vi "test_libssh2_channel_forward_accept.vi"() -> ()   [LabVIEW 2013, in "libssh2_integration_tests.lvlib"]
uses:
  libssh2_integration_tests.lvlib
  <vilib>/addons/_JKI Toolkits/Caraya/classes/Test/Test.lvclass
  support/support.lvlib
  libssh2/libssh2.lvlib
  <vilib>/addons/_JKI Toolkits/Caraya/classes/Assert/Assert.lvclass
panel:
  out "error out":errorcluster
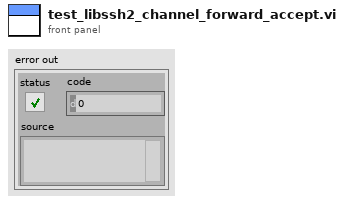
[diagram p1: front panel]
types:
  T1 = typedef "libssh2.lvlib/Session Refnum.ctl" = refnum<k1>
  T2 = typedef "libssh2.lvlib/Listener Refnum.ctl" = refnum<k1>
  T3 = typedef "libssh2.lvlib/Channel Refnum.ctl" = refnum<k1>
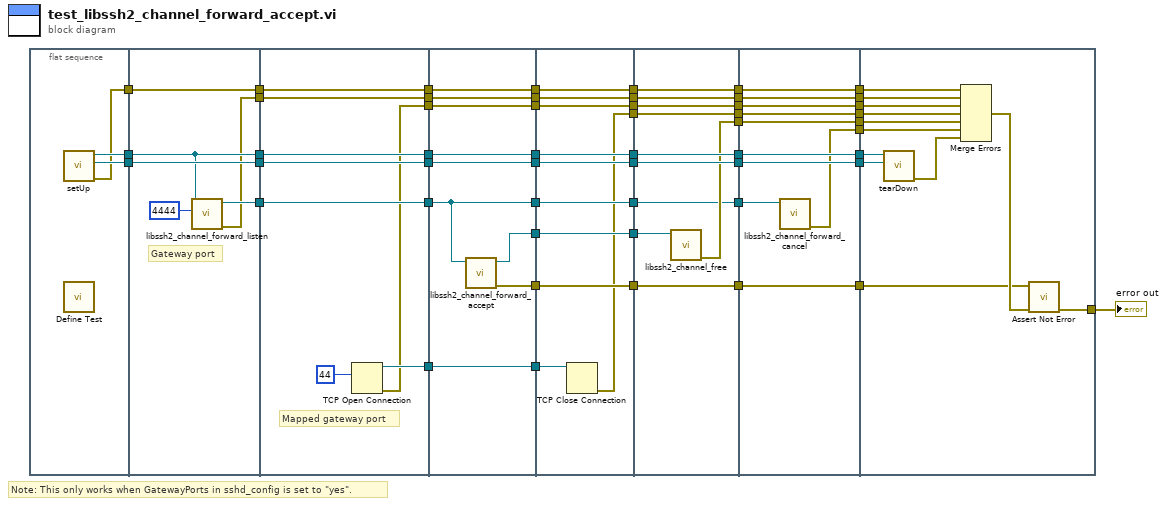
[diagram p0: block diagram]
diagram:
  # "Note: This only works when GatewayPorts in sshd_config is set to \"yes\"."
  n1 = flat-sequence {
    tunnel: [w55] -> w52
    tunnel: [w54] -> w51
    tunnel: [w53] -> w50
    tunnel: w52 -> [w59]
    tunnel: w51 -> [w61]
    tunnel: [w59] -> w33
    tunnel: [w61] -> w31
    tunnel: w50 -> [w60]
    tunnel: [w60] -> w29
    tunnel: [w57] -> w27
    tunnel: [w58] -> w25
    tunnel: w33 -> [w65]
    tunnel: [w65] -> w32
    tunnel: w31 -> [w69]
    tunnel: [w69] -> w30
    tunnel: w29 -> [w68]
    tunnel: [w68] -> w28
    tunnel: w27 -> [w67]
    tunnel: [w67] -> w26
    tunnel: w25 -> [w66]
    tunnel: [w66] -> w24
    tunnel: [w63] -> w23
    tunnel: [w62] -> w22
    tunnel: w32 -> [w78]
    tunnel: [w78] -> w43
    tunnel: w30 -> [w77]
    tunnel: [w77] -> w42
    tunnel: w28 -> [w76]
    tunnel: [w76] -> w41
    tunnel: w26 -> [w75]
    tunnel: [w75] -> w40
    tunnel: w24 -> [w74]
    tunnel: [w74] -> w39
    tunnel: [w73] -> w38
    tunnel: [w71] -> w37
    tunnel: [w72] -> w35
    tunnel: w23 -> [w71]
    tunnel: w22 -> [w70]
    tunnel: [w70] -> w21
    tunnel: w43 -> [w88]
    tunnel: w42 -> [w87]
    tunnel: [w88] -> w49
    tunnel: [w87] -> w48
    tunnel: [w84] -> w47
    tunnel: w41 -> [w86]
    tunnel: [w86] -> w46
    tunnel: w40 -> [w85]
    tunnel: [w85] -> w45
    tunnel: w39 -> [w81]
    tunnel: w38 -> [w84]
    tunnel: w37 -> [w82]
    tunnel: [w83] -> w36
    tunnel: w35 -> [w83]
    tunnel: [w81] -> w34
    tunnel: w21 -> [w80]
    tunnel: [w80] -> w20
    tunnel: [w79] -> w19
    tunnel: w49 -> [w98]
    tunnel: w48 -> [w97]
    tunnel: w47 -> [w96]
    tunnel: [w98] -> w18
    tunnel: [w97] -> w16
    tunnel: [w95] -> w14
    tunnel: w46 -> [w94]
    tunnel: [w94] -> w12
    tunnel: w45 -> [w93]
    tunnel: [w93] -> w10
    tunnel: [w92] -> w8
    tunnel: w36 -> [w92]
    tunnel: [w91] -> w6
    tunnel: w34 -> [w91]
    tunnel: w20 -> [w90]
    tunnel: [w90] -> w5
    tunnel: w19 -> [w89]
    tunnel: [w89] -> w3
    tunnel: w18 -> [w108]
    tunnel: [w108] -> w17
    tunnel: w16 -> [w107]
    tunnel: [w107] -> w15
    tunnel: w14 -> [w106]
    tunnel: [w106] -> w13
    tunnel: w12 -> [w105]
    tunnel: [w105] -> w11
    tunnel: w10 -> [w104]
    tunnel: [w104] -> w9
    tunnel: w8 -> [w103]
    tunnel: [w103] -> w7
    tunnel: w6 -> [w100]
    tunnel: w5 -> [w102]
    tunnel: [w102] -> w4
    tunnel: w3 -> [w101]
    tunnel: [w101] -> w2
    tunnel: [w99] -> w1
    tunnel: w17 -> [w120]
    tunnel: w15 -> [w119]
    tunnel: [w118] -> w44
    tunnel: w13 -> [w116]
    tunnel: w11 -> [w115]
    tunnel: w9 -> [w113]
    tunnel: w7 -> [w112]
    tunnel: w4 -> [w111]
    tunnel: w2 -> [w110]
    tunnel: w1 -> [w109]
    frame #0 {
      n2 = call "setUp.vi"() -> ("error out"=w53:errorcluster, "connection ID"=w54:refnum<k5>, "session"=w55:T1)  [unwired: 9 in]
      n3 = call <vilib>:"Define Test.vi"() -> ()  [unwired: 10 in, 2 out]
    }
    frame #1 {
      # "Gateway port"
      n4 = call "libssh2_channel_forward_listen.vi"("port in"=4444, "session"=w59) -> ("error out"=w57:errorcluster, "listener"=w58:T2)  [unwired: 7 in, 1 out]
    }
    frame #2 {
      # "Mapped gateway port"
      n5 = TCP Open Connection(remote port or service name=u16 44) -> (connection ID=w63:refnum<k5>, error out=w62:errorcluster)  [unwired: 4 in]
    }
    frame #3 {
      n6 = call "libssh2_channel_forward_accept.vi"("listener"=w74) -> ("error out"=w72:errorcluster, "channel"=w73:T3)  [unwired: 9 in]
    }
    frame #4 {
      n7 = TCP Close Connection(connection ID=w82) -> (error out=w79:errorcluster)  [unwired: 2 in, 1 out]
    }
    frame #5 {
      n8 = call "libssh2_channel_free.vi"("channel"=w96) -> ("error out"=w95:errorcluster)  [unwired: 10 in]
    }
    frame #6 {
      n9 = call "libssh2_channel_forward_cancel.vi"("listener"=w100) -> ("error out"=w99:errorcluster)  [unwired: 10 in]
    }
    frame #7 {
      n10 = call "tearDown.vi"("connection ID"=w119, "session"=w120) -> ("error out"=w117:errorcluster)  [unwired: 9 in]
      n11 = Merge Errors(w115, w113, w111, w110, w116, w109, w117) -> (w114:errorcluster)
      n12 = call <vilib>:"Assert Not Error.vi"("error in (no error)"=w114, "Not Error?"=w112) -> ("error out"=w118:errorcluster)  [unwired: 8 in, 1 out]
    }
  }
  "error out" <- w44
